vi "Processing Step.vi"(8 "error in (no error)":errorcluster, 11 "Connection Handler in":refnum<class "Connection Handler.lvclass">) -> (0 "error out":errorcluster, 2 "Processing Step":T1, 3 "Connection Handler out":refnum<class "Connection Handler.lvclass">)   [LabVIEW 2020, in "HTTP Server.lvlib" / "Connection Handler.lvclass"]
uses:
  Connection Handler.lvclass
  Processing Step.ctl
  HTTP Server.lvlib
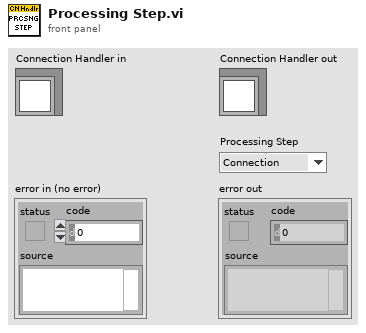
[diagram p1: front panel]
types:
  T1 = typedef "HTTP Server.lvlib/Processing Step.ctl" = enum16{"Connection", "Request", "Routing", "Controller Init", "Controller", "Response", "Cleanup", "Exception"}
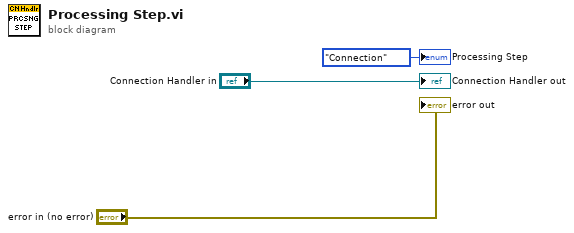
[diagram p0: block diagram]
diagram:
  "error out" <- "error in (no error)"
  "Connection Handler out" <- "Connection Handler in"
  "Processing Step" <- Processing_Step."Connection" ("Processing Step")
